vi "SVT Gain and Phase (Time).vi"(0 "stimulus signal X [EUx]":waveform(dbl), 1 "response signal Y [EUy]":waveform(dbl), 3 "advanced span [Hz]":dbl=-1.0 format="%.2f", 5 "error in (no error)":errorcluster, 6 "desired units":T9, 9 "expected fundamental frequency [Hz]":dbl=-1.0 format="%.2f") -> (11 "detected tone response":cluster{"frequency [Hz]":dbl, "amplitude":dbl}={"frequency [Hz]"=nan, "amplitude"=nan} {"amplitude" format="%.3f"; "frequency [Hz]" format="%.2f"}, 12 "unit labels":T8, 13 "detected tone stimulus":cluster{"frequency [Hz]":dbl, "amplitude":dbl}={"frequency [Hz]"=nan, "amplitude"=nan} {"amplitude" format="%.3f"; "frequency [Hz]" format="%.2f"}, 14 "complex spectrum\nstimulus X":T7={"complex spectrum response"={"f0"=0.0, "df"=1.0, "complex spectrum"=[]}, "spectrum info"={"channel name"="", "description"="", "x-axis units"=0, "spectral info"={"spectrum type"=enum."Power [Magnitude^2]", "linear/dB"=enum."linear", "window"=0, "window size"=0, "FFT size"=0}, "engineering units"=0, "custom label"="", "dB reference [EU]"=0.0, "peak units"=enum."rms", "weighting filter"=0, "spectral density?"=FALSE, "unit label"="", "spectrum skewed?"=FALSE, "complimentary spectrum units"=enum."none"}} {"spectrum info"."x-axis units" items=["Time (s)"=0, "Frequency-CB (Hz)"=1, "Frequency-CPB (Hz)"=1248, "Frequency-Arbitrary (Hz)"=2357, "Quefrency (s)"=2, "Revolutions (rev)"=3, "Order"=4, "Speed (RPM)"=11, "Speed (rad/s)"=21, "Index"=65535]; "spectrum info"."weighting filter" items=["Linear", "A-weighting", "B-weighting", "C-weighting", "ITU-R 468-4", "Dolby", "CCITT", "C-message", "Wb", "Wc", "Wd", "We", "Wf", "Wh", "Wj", "Wk", "Wm", "AES17 20 kHz lowpass", "AES17 40 kHz lowpass", "AES17 20 kHz highpass", "AES17 40 kHz highpass"]; "spectrum info"."dB reference [EU]" format="%.2f"; "spectrum info"."engineering units" items=["custom..."=0, "V"=1, "A"=21, "C"=30, "pC"=31, "s"=32, "-"=29, "Pa"=2, "N"=20, "g"=3, "m/s^2"=4, "m/s"=5, "m"=6, "mm/s"=12, "mm"=13, "micron/s"=14, "micron"=15, "in/s^2"=7, "in/s"=8, "in"=9, "mil/s"=10, "mil"=11, "rad/s^2"=16, "rad/s"=17, "rad"=18, "deg/s^2"=26, "deg/s"=27, "deg"=28, "RPM"=22, "cycle/s^2"=23, "Hz"=24, "cycle"=25, "strain"=19]; "spectrum info"."spectral info"."window" items=["None "=0, "Hanning"=1, "Hamming"=2, "Blackman-Harris"=3, "Exact Blackman"=4, "Blackman"=5, "Flat Top"=6, "4 Term B-Harris "=7, "7 Term B-Harris"=8, "Low Sidelobe"=9, "Force - Exponential"=10, "Gaussian"=62]; "complex spectrum response"."complex spectrum" format="%.2f"; "complex spectrum response"."df" format="%.2f"; "complex spectrum response"."f0" format="%.2f"}, 15 "complex spectrum\nresponse Y":T7={"complex spectrum response"={"f0"=0.0, "df"=1.0, "complex spectrum"=[]}, "spectrum info"={"channel name"="", "description"="", "x-axis units"=0, "spectral info"={"spectrum type"=enum."Power [Magnitude^2]", "linear/dB"=enum."linear", "window"=0, "window size"=0, "FFT size"=0}, "engineering units"=0, "custom label"="", "dB reference [EU]"=0.0, "peak units"=enum."rms", "weighting filter"=0, "spectral density?"=FALSE, "unit label"="", "spectrum skewed?"=FALSE, "complimentary spectrum units"=enum."none"}} {"spectrum info"."x-axis units" items=["Time (s)"=0, "Frequency-CB (Hz)"=1, "Frequency-CPB (Hz)"=1248, "Frequency-Arbitrary (Hz)"=2357, "Quefrency (s)"=2, "Revolutions (rev)"=3, "Order"=4, "Speed (RPM)"=11, "Speed (rad/s)"=21, "Index"=65535]; "spectrum info"."weighting filter" items=["Linear", "A-weighting", "B-weighting", "C-weighting", "ITU-R 468-4", "Dolby", "CCITT", "C-message", "Wb", "Wc", "Wd", "We", "Wf", "Wh", "Wj", "Wk", "Wm", "AES17 20 kHz lowpass", "AES17 40 kHz lowpass", "AES17 20 kHz highpass", "AES17 40 kHz highpass"]; "spectrum info"."dB reference [EU]" format="%.2f"; "spectrum info"."engineering units" items=["custom..."=0, "V"=1, "A"=21, "C"=30, "pC"=31, "s"=32, "-"=29, "Pa"=2, "N"=20, "g"=3, "m/s^2"=4, "m/s"=5, "m"=6, "mm/s"=12, "mm"=13, "micron/s"=14, "micron"=15, "in/s^2"=7, "in/s"=8, "in"=9, "mil/s"=10, "mil"=11, "rad/s^2"=16, "rad/s"=17, "rad"=18, "deg/s^2"=26, "deg/s"=27, "deg"=28, "RPM"=22, "cycle/s^2"=23, "Hz"=24, "cycle"=25, "strain"=19]; "spectrum info"."spectral info"."window" items=["None "=0, "Hanning"=1, "Hamming"=2, "Blackman-Harris"=3, "Exact Blackman"=4, "Blackman"=5, "Flat Top"=6, "4 Term B-Harris "=7, "7 Term B-Harris"=8, "Low Sidelobe"=9, "Force - Exponential"=10, "Gaussian"=62]; "complex spectrum response"."complex spectrum" format="%.2f"; "complex spectrum response"."df" format="%.2f"; "complex spectrum response"."f0" format="%.2f"}, 16 "gain":dbl=nan format="%.2f", 17 "phase lag":dbl=nan format="%.2f", 19 "error out":errorcluster)   [LabVIEW 2017, in "SoundVib_SingleTone.lvlib"]
doc: "Computes the gain and phase between <B>stimulus signal X</B> and <B>response signal Y</B> at the fundamental frequency. This VI returns the detected fundamental frequency, detected response amplitude, gain, and phase lag. This VI does not maintain state internally; you can use this VI in a loop to process multiple blocks. Wire data to the <B>stimulus signal X [Eux]</B> and <B>response signal Y [Euy]</B> inputs to determine the polymorphic instance to use or manually select the instance."
uses:
  <vilib>/addons/Sound and Vibration/svt_Single Tone Measurements/SoundVib_SingleTone.lvlib
  <vilib>/addons/_NISVFA/_Shared subVIs/Controls/svc_Spectrum Info.ctl
  <vilib>/addons/_NISVFA/_Shared subVIs/Controls/svc_X-Axis Units.ctl
  <vilib>/addons/_NISVFA/_Shared subVIs/Controls/svc_Spectrum Type.ctl
  <vilib>/addons/_NISVFA/_Shared subVIs/Controls/svc_Engineering Units Text Ring.ctl
  <vilib>/addons/_NISVFA/_Shared subVIs/Controls/svc_Weighting Filter Text Ring.ctl
  <vilib>/addons/_NISVFA/_Shared subVIs/Controls/svc_Complimentary Spectrum Units.ctl
  <vilib>/addons/_NISVFA/_Shared subVIs/Controls/svc_Window.ctl
  <vilib>/addons/Sound and Vibration/svt_Distortion/SoundVib_Distortion.lvlib
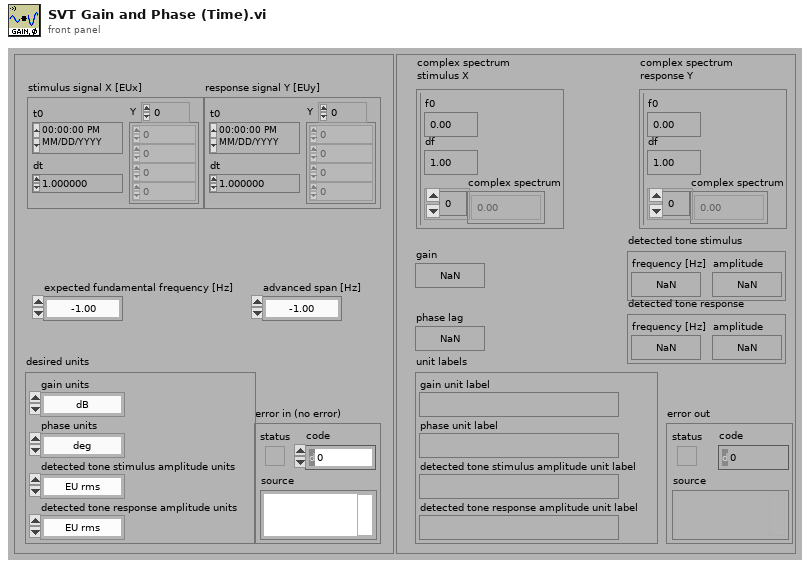
[diagram p1: front panel]
types:
  T1 = typedef "svc_Spectrum Info.ctl" = cluster{"channel name":string, "description":string, "x-axis units":T2, "spectral info":cluster{"spectrum type":T3, "linear/dB":enum16{"linear", "dB"}, "window":u16, "window size":i32, "FFT size":i32}, "engineering units":T4, "custom label":string, "dB reference [EU]":dbl, "peak units":enum16{"rms", "peak", "peak-peak"}, "weighting filter":T5, "spectral density?":bool, "unit label":string, "spectrum skewed?":bool, "complimentary spectrum units":T6}
  T2 = typedef "svc_X-Axis Units.ctl" = u16
  T3 = typedef "svc_Spectrum Type.ctl" = enum16{"FFT Spectrum [complex]", "Amplitude [Magnitude]", "Power [Magnitude^2]", "Cross Spectrum [complex]", "Frequency Response [Complex]"}
  T4 = typedef "svc_Engineering Units Text Ring.ctl" = u16
  T5 = typedef "svc_Weighting Filter Text Ring.ctl" = u16
  T6 = typedef "svc_Complimentary Spectrum Units.ctl" = enum16{"none", "radians", "degrees", "cycles", "imaginary"}
  T7 = cluster{"complex spectrum response":cluster{"f0":dbl, "df":dbl, "complex spectrum":cdb[]}, "spectrum info":T1}
  T8 = cluster{"gain unit label":string, "phase unit label":string, "detected tone stimulus amplitude unit label":string, "detected tone response amplitude unit label":string}
  T9 = cluster{"gain units":enum16{"dB", "linear ratio"}, "phase units":enum16{"deg", "rad"}, "detected tone stimulus amplitude units":enum16{"EU rms", "EU peak", "EU peak-peak"}, "detected tone response amplitude units":enum16{"EU rms", "EU peak", "EU peak-peak"}}
  T10 = cluster{"gain unit label":string, "phase unit label":string, "detected tone stimulus unit label":string, "detected response stimulus unit label":string}
  T11 = typedef "svc_Window.ctl" = u32
  T12 = cluster{"complex spectrum":cluster{"f0":dbl, "df":dbl, "complex spectrum":cdb[]}, "spectrum info":T1}
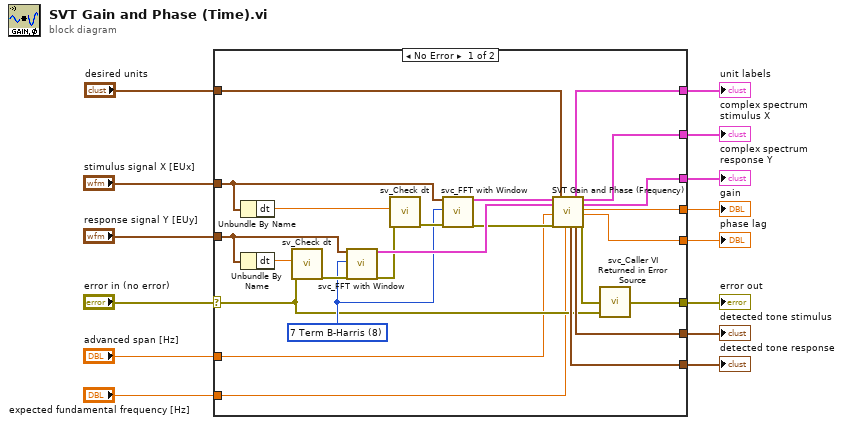
[diagram p0: block diagram]
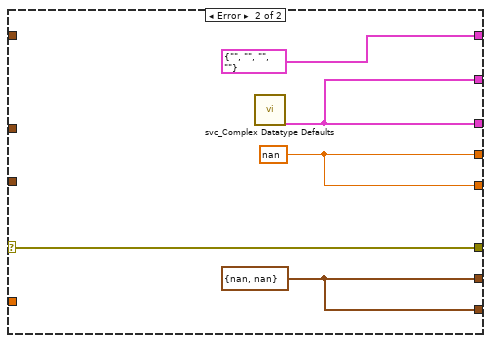
[diagram p2: hidden frame]
diagram:
  n1 = case shown="No Error" "error in (no error)" {
    selector: "error in (no error)" -> [w17 w43]
    tunnel: "response signal Y [EUy]" -> [w19 _]
    tunnel: "stimulus signal X [EUx]" -> [w18 _]
    tunnel: [w29 w43] -> w12
    tunnel: [w38 w42] -> w11
    tunnel: [w37 w42] -> w9
    tunnel: [w27 w39] -> w4
    tunnel: [w33 w41] -> w8
    tunnel: [w34 w41] -> w7
    tunnel: "desired units" -> [w32 _]
    tunnel: [w31 T10 {"gain unit label"="", "phase unit label"="", "detected tone stimulus unit label"="", "detected response stimulus unit label"=""} ("unit labels")] -> w5
    tunnel: [w26 w39] -> w3
    tunnel: "expected fundamental frequency [Hz]" -> [w16 _]
    tunnel: "advanced span [Hz]" -> [w15 _]
    frame No Error {
      w22 = T11 8 items=["None ", "Hanning", "Hamming", "Blackman-Harris", "Exact Blackman", "Blackman", "Flat Top", "4 Term B-Harris ", "7 Term B-Harris", "Low Sidelobe"] ("window")
      n2 = Unbundle By Name(w18) -> ("dt"=w21:dbl)
      n3 = Unbundle By Name(w19) -> ("dt"=w20:dbl)
      n4 = call <vilib>:"sv_Check dt.vi"("error in"=w17, "dt"=w20) -> ("error out"=w25:errorcluster)  [unwired: 8 in, 1 out]
      n5 = call <vilib>:"svc_FFT with Window.vi"("time signal in [EU]"=w19, "window"=w22, "error in (no error)"=w25) -> ("complex spectrum"=w35:T7, "error out"=w24:errorcluster)  [unwired: 15 in]
      n6 = call <vilib>:"sv_Check dt.vi"("error in"=w24, "dt"=w21) -> ("error out"=w23:errorcluster)  [unwired: 8 in, 1 out]
      n7 = call <vilib>:"svc_FFT with Window.vi"("time signal in [EU]"=w18, "window"=w22, "error in (no error)"=w23) -> ("complex spectrum"=w36:T7, "error out"=w28:errorcluster)  [unwired: 15 in]
      n8 = call <vilib>:"SVT Gain and Phase (Frequency).vi"("complex spectrum\nstimulus X"=w36, "complex spectrum\nresponse Y"=w35, "advanced span [Hz]"=w15, "error in (no error)"=w28, "desired units"=w32, "expected fundamental frequency [Hz]"=w16) -> ("detected tone response"=w33:cluster{"frequency [Hz]":dbl, "amplitude":dbl}, "unit labels"=w31:T8, "detected tone stimulus"=w34:cluster{"frequency [Hz]":dbl, "amplitude":dbl}, "dup complex spectrum\nstimulus X"=w26:T7, "dup complex spectrum\nresponse Y"=w27:T7, "gain"=w37:dbl, "phase lag"=w38:dbl, "error out"=w30:errorcluster)  [unwired: 6 in]
      n9 = call <vilib>:"svc_Caller VI Returned in Error Source.vi"("warning input to caller"=w17, "error in (no error)"=w30) -> ("error out"=w29:errorcluster)  [unwired: 3 in]
    }
    frame Error {
      w41 = cluster{"frequency [Hz]":dbl, "amplitude":dbl} {"frequency [Hz]"=nan, "amplitude"=nan} ("detected tone stimulus")
      w42 = nan ("phase lag")
      n10 = call <vilib>:"svc_Complex Datatype Defaults.vi"() -> ("complex spectrum"=w39:T12)  [unwired: 11 in, 8 out]
    }
  }
  "phase lag" <- w11
  "error out" <- w12
  "gain" <- w9
  "complex spectrum\nresponse Y" <- w4
  "unit labels" <- w5
  "detected tone response" <- w8
  "detected tone stimulus" <- w7
  "complex spectrum\nstimulus X" <- w3
